vi "Write session reservation in.vi"(0 "AbstractDMM in":refnum<class "Abstract_Instrument.lvclass">, 5 "MeasurementLink Session Management V1.lvlib:Session Reservation.lvclass":refnum<class "Session Reservation.lvclass">, 11 "error in (no error)":errorcluster) -> (4 "AbstractDMM out":refnum<class "Abstract_Instrument.lvclass">, 15 "error out":errorcluster)   [LabVIEW 2020, in "Abstract_Instrument.lvlib" / "Abstract_Instrument.lvclass"]
uses:
  Abstract_Instrument.lvclass
  <vilib>/MeasurementLink/MeasurementLink Session Management V1/Session Reservation/Session Reservation.lvclass
  Abstract_Instrument.lvclass/Abstract_Instrument.ctl
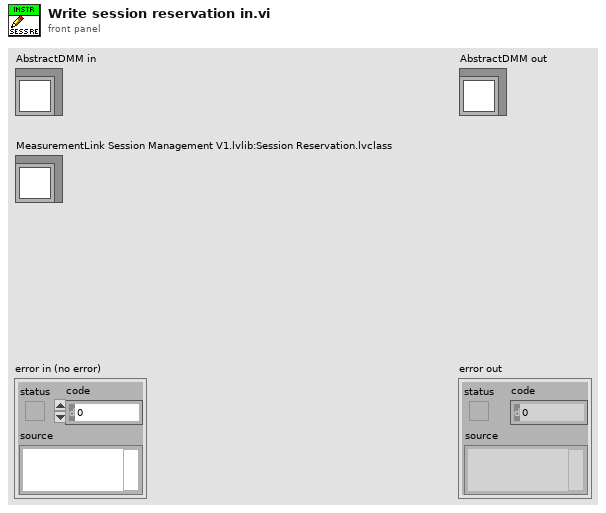
[diagram p1: front panel]
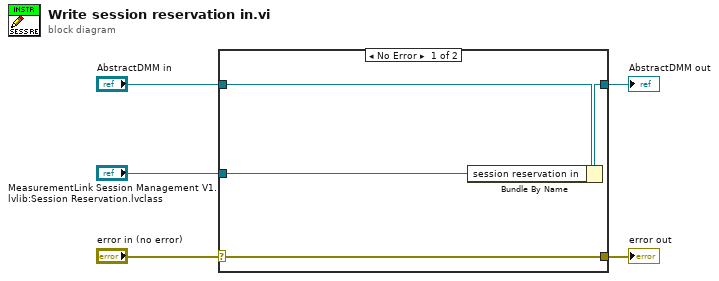
[diagram p0: block diagram]
diagram:
  n1 = case shown="No Error" "error in (no error)" {
    selector: "error in (no error)" -> [w9 w10]
    tunnel: [w9 w10] -> w4
    tunnel: [w7 w11] -> w2
    tunnel: "AbstractDMM in" -> [w8 w11]
    tunnel: "MeasurementLink Session Management V1.lvlib:Session Reservation.lvclass" -> [w6 _]
    frame No Error {
      n2 = Bundle By Name(cluster=w8, "session reservation in"=w6) -> (w7:refnum<class "Abstract_Instrument.lvclass">)
    }
    frame Error {
    }
  }
  "error out" <- w4
  "AbstractDMM out" <- w2
